vi "Get Relay Names.vi"(8 "error in (no error)":errorcluster, 11 "session in":T1) -> (0 "error out":errorcluster, 2 "relay names":string[](array[string]), 3 "session out":T1)   [LabVIEW 2020, in "SLSC Switch.lvlib"]
doc: "Returns a string array of valid relay names for the NI-SLSC Switch module."
uses:
  <vilib>/SLSC_Switch/SLSC Switch.lvlib
  nislscsl.dll
  <vilib>/userdefined/High Color/SLSC_Switch/nislscslSession.ctl
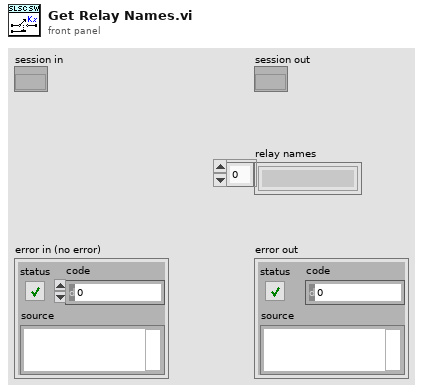
[diagram p1: front panel]
types:
  T1 = typedef "nislscslSession.ctl" = refnum<k20>
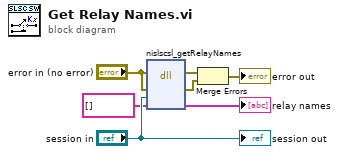
[diagram p0: block diagram]
diagram:
  n1 = dll-call lib="nislscsl.*" fn="nislscsl_getRelayNames"(error in="error in (no error)", "errorCluster"="error in (no error)", "sessionHandle"="session in", "relayNames"=string[] [] ("array of strings")) -> (error out=w7:errorcluster, "errorCluster"=w6:errorcluster, "relayNames"=→"relay names":string[])  [unwired: 4 in, 1 out]
  n2 = Merge Errors(w7, w6) -> (→"error out":errorcluster)
  "session out" <- "session in"
